vi "GEA2 Disconnect Handling.vi"() -> ()   [LabVIEW 2016]
uses:
  Q:/Common/LabVIEW GEA2 Toolkit/LabVIEW_GEA2_Toolkit.lvlibp/type defs/ERD Read Data In.ctl
  Q:/Common/LabVIEW GEA2 Toolkit/LabVIEW_GEA2_Toolkit.lvlibp/type defs/Data Type.ctl
  Q:/Common/LabVIEW GEA2 Toolkit/LabVIEW_GEA2_Toolkit.lvlibp/type defs/Source_Destination.ctl
  Q:/Common/LabVIEW GEA2 Toolkit/LabVIEW_GEA2_Toolkit.lvlibp
panel:
  out "Boolean":bool
  in  "Stop Button":bool
  out "Data":string
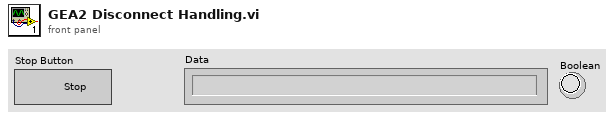
[diagram p1: front panel]
types:
  T1 = typedef "LabVIEW_GEA2_Toolkit.lvlibp/Source_Destination.ctl" = cluster{"Source":u8, "Destination":u8}
  T2 = typedef "LabVIEW_GEA2_Toolkit.lvlibp/ERD Read Data In.ctl" = cluster{"ERD Number":u16, "Data Type":T3}
  T3 = typedef "LabVIEW_GEA2_Toolkit.lvlibp/Data Type.ctl" = enum16{"string", "boolean", "uint8_t", "uint16_t", "uint32_t", "uint64_t", "int8_t", "int16_t", "int32_t", "int64_t"}
  T4 = typedef "LabVIEW_GEA2_Toolkit.lvlibp/ERD Read Data Out.ctl" = cluster{"ERD Number":u16, "Data":string}
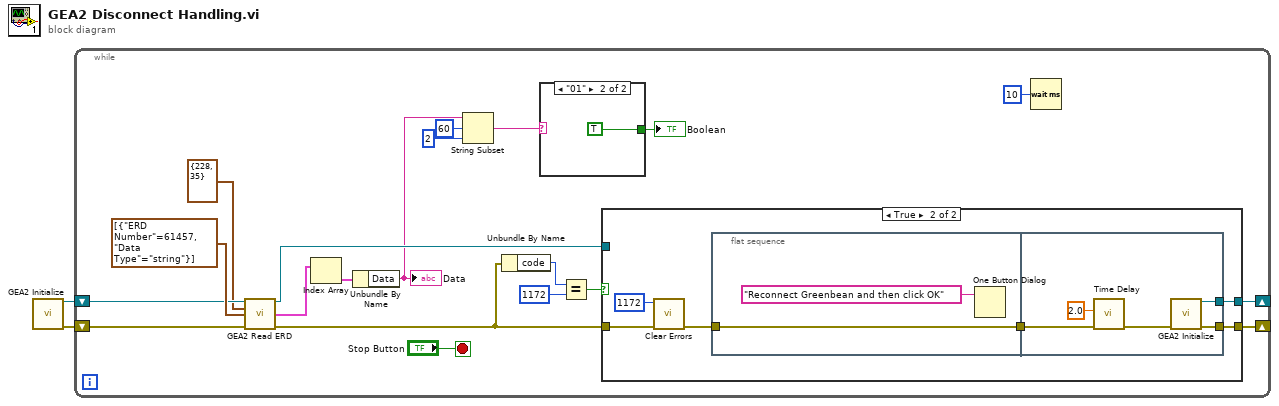
[diagram p0: block diagram]
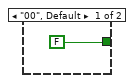
[diagram p2: hidden frame]
diagram:
  n1 = call "GEA2 Initialize.vi"() -> ("GEA2 Reference Out"=w1:refnum<k24>, "error out"=w2:errorcluster)  [unwired: 13 in, 1 out]
  n2 = while {
    shift-right: [w8] -> _
    shift-left: w1 -> [w20]
    shift-right: [w9] -> _
    shift-left: w2 -> [w22]
    stop <- "Stop Button" stop-if-true
    n3 = call "GEA2 Read ERD.vi"("GEA2 Reference In"=w20, "GEA Inputs"=T1 {"Source"=228, "Destination"=35}, "Read ERD List"=T2[] [{"ERD Number"=61457, "Data Type"=enum."string"}], "Error In"=w22) -> ("GEA2 Reference Out"=w10:refnum<k24>, "ERD Data Out"=w18:T4[], "Error Out"=w11:errorcluster)  [unwired: 8 in, 1 out]
    n4 = Index Array(array=w18) -> (element=w17:T4)  [unwired: 1 in]
    n5 = Unbundle By Name(w17) -> ("Data"=w7:string)
    "Data" <- w7
    n6 = String Subset(string=w7, offset (0)=60, length (rest)=2 ("length (rest)")) -> (substring=w4:string)
    n7 = Unbundle By Name(w11) -> ("code"=w14:i32)
    n8 = case shown="\"01\"" w4 {
      tunnel: [FALSE TRUE] -> w3
      frame "00", Default {
      }
      frame "01" {
      }
    }
    "Boolean" <- w3
    n9 = Equal?(x=w14, y=1172) -> (x = y?=w12:bool)
    n10 = case shown="True" w12 {
      tunnel: w11 -> [w25 w30]
      tunnel: [w26 w32] -> w8
      tunnel: w10 -> [w26 _]
      tunnel: [w25 w31] -> w9
      frame False {
      }
      frame True {
        n11 = call <vilib>:"Clear Errors.vi"("error in (no error)"=w30, "specific error code to clear (0: all)"=1172) -> ("error out"=w29:errorcluster)  [unwired: 4 in, 1 out]
        n12 = flat-sequence {
          tunnel: w29 -> [w34]
          tunnel: [w34] -> w27
          tunnel: [w39] -> w32
          tunnel: [w38] -> w31
          tunnel: w27 -> [w37]
          frame #0 {
            n13 = One Button Dialog(message="Reconnect Greenbean and then click OK") -> ()  [unwired: 1 in, 1 out]
          }
          frame #1 {
            n14 = call "Time Delay"("error in (no error)"=w37, "Delay Time (s)"=2.0) -> ("error out"=w36:errorcluster)  [unwired: 9 in]
            n15 = call "GEA2 Initialize.vi"("error in"=w36) -> ("GEA2 Reference Out"=w39:refnum<k24>, "error out"=w38:errorcluster)  [unwired: 12 in, 1 out]
          }
        }
      }
    }
    n16 = Wait (ms)(milliseconds to wait=u32 10) -> ()  [unwired: 1 out]
  }
